vi "Write.vi"(8 "error in (no error)":errorcluster, 9 "Start address":string, 10 "Read Type":variant, 11 "MelsecTCP in":refnum<class "Abs Controler.lvclass">) -> (0 "error out":errorcluster, 3 "MelsecTCP out":refnum<class "Abs Controler.lvclass">)   [LabVIEW 2020, in "HslCommunication.lvlib" / "Abs Controler.lvclass"]
uses:
  Abs Controler.lvclass
  E:/Git/Libraries/develop/HslCommunication/_Dependenciecs/HslCommunication.dll
  _Dependenciecs/HslCommunication.dll
  <vilib>/Utility/Data Type/NI_Data Type.lvlib
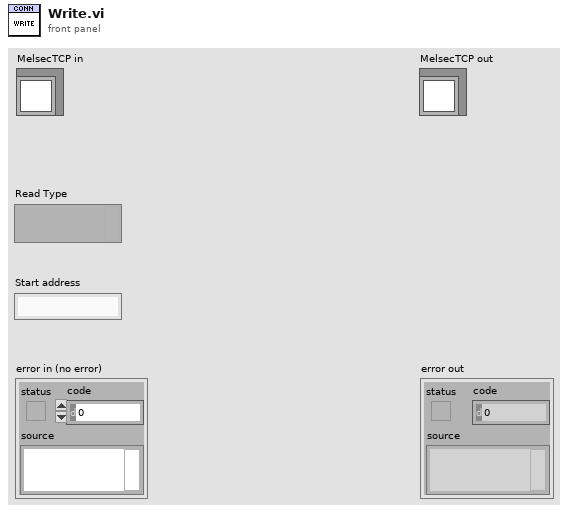
[diagram p1: front panel]
types:
  T1 = typedef "NI_Data Type.lvlib/Data Type.ctl" = enum8{"Invalid Type", "Void", "I8", "I16", "I32", "I64", "U8", "U16", "U32", "U64", "Single Float", "Double Float", "Extended Float", "Single Complex", "Double Complex", "Extended Complex", "Enum U8", "Enum U16", "Enum U32", "Enum U64", "Single Float With Unit", "Double Float With Unit", "Extended Float With Unit", "Single Complex with Unit", "Double Complex with Unit", "Extended Complex with Unit", "Boolean", "String", "Path", "Picture", "Tag", "Array", "Cluster", "Variant", "LV Variant", "Waveform", "Timestamp", "Digital Waveform", "Digital Data", "ExpressData", "Refnum", "External Data", "VI", "Poly VI", "LabVIEW Class Instance", "Fixed Point", "Set Collection", "Map Collection"}
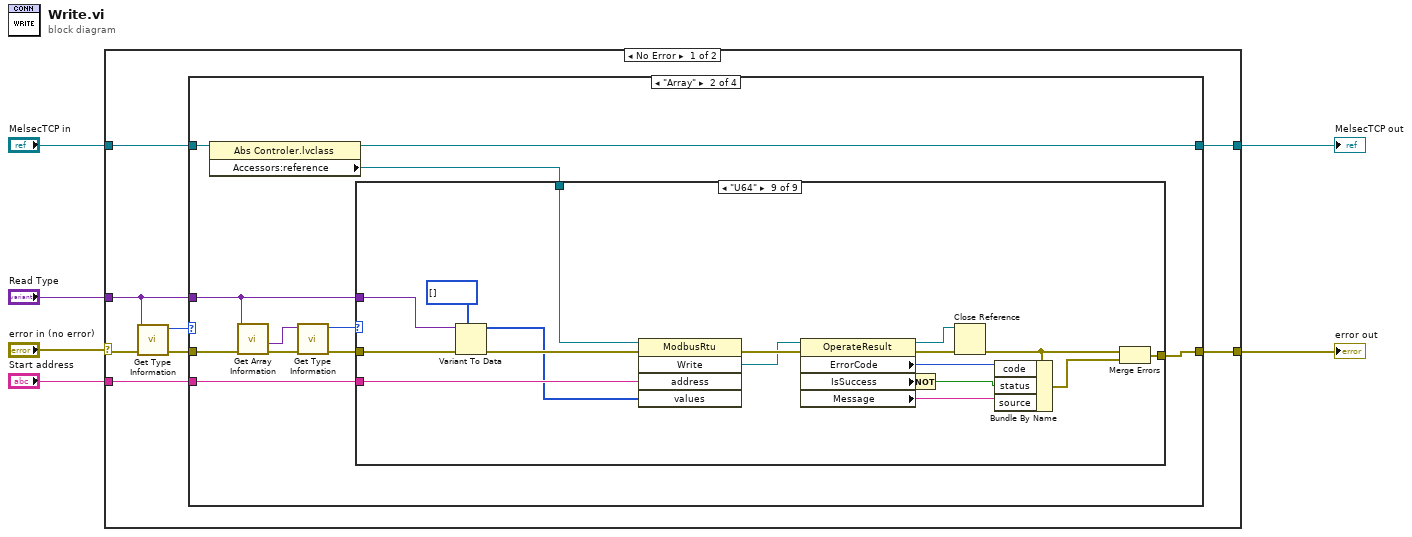
[diagram p0: block diagram]
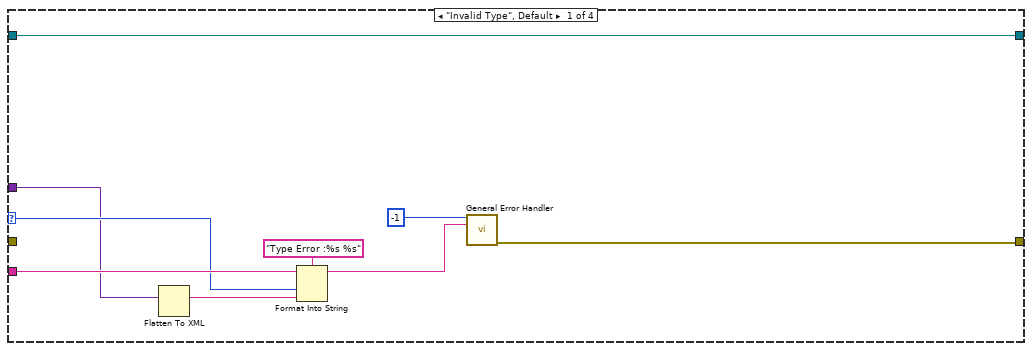
[diagram p2: hidden frame]
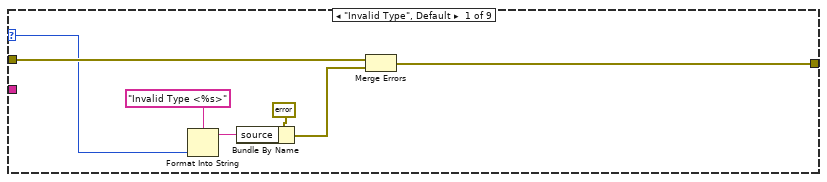
[diagram p3: hidden frame]
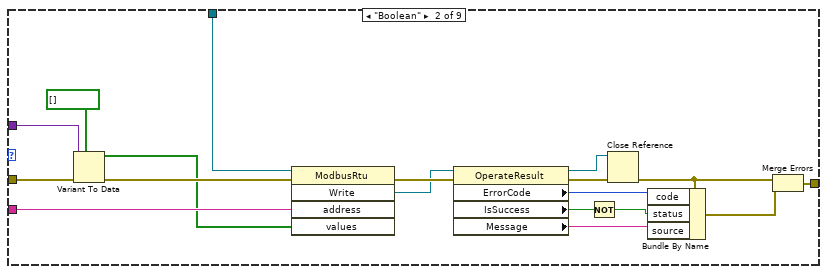
[diagram p4: hidden frame]
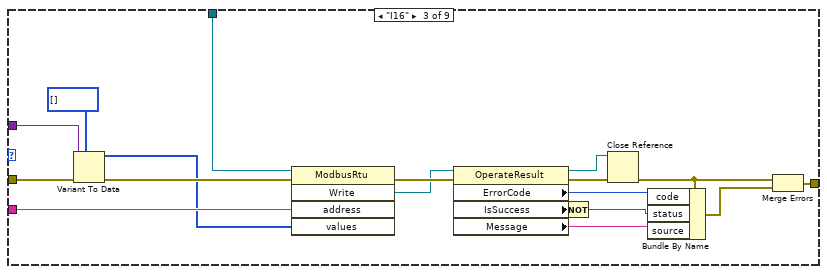
[diagram p5: hidden frame]
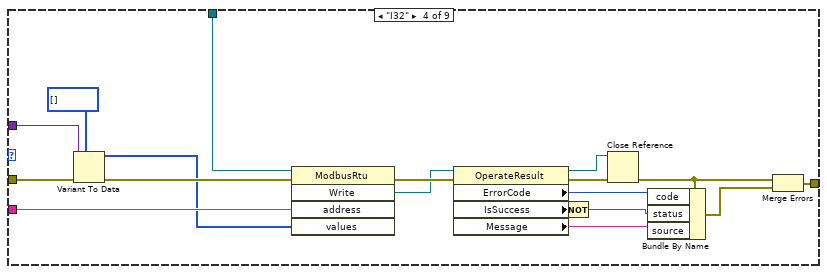
[diagram p6: hidden frame]
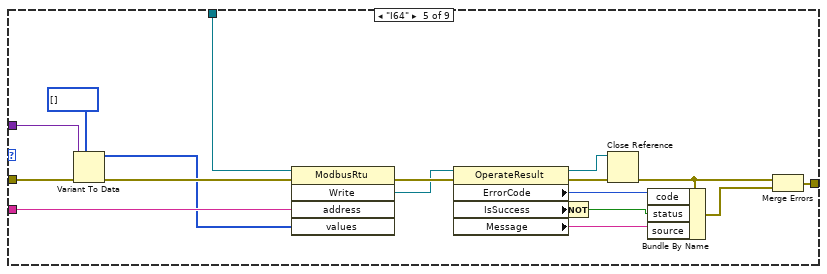
[diagram p7: hidden frame]
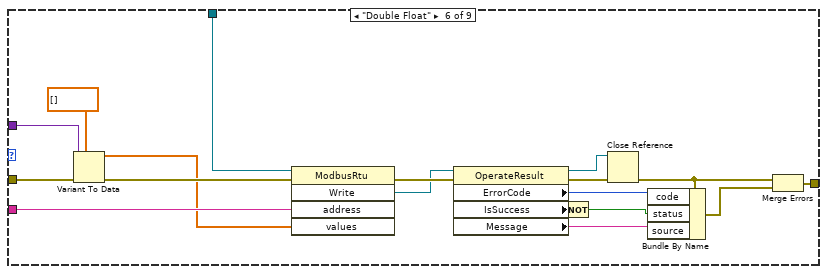
[diagram p8: hidden frame]
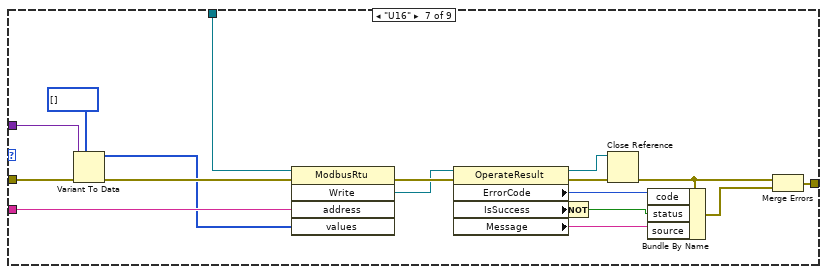
[diagram p9: hidden frame]
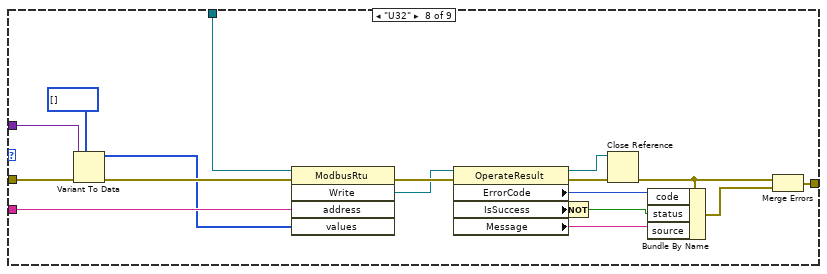
[diagram p10: hidden frame]
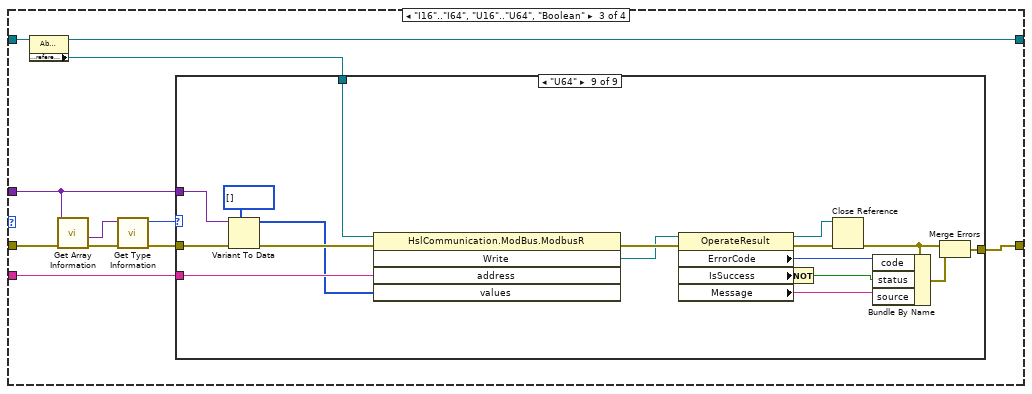
[diagram p11: hidden frame]
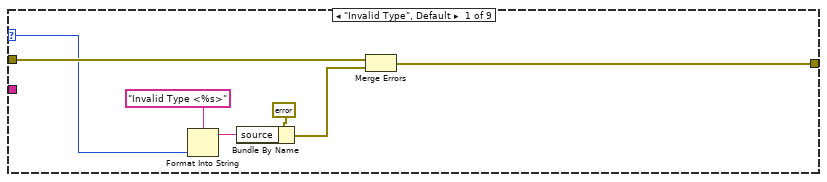
[diagram p12: hidden frame]
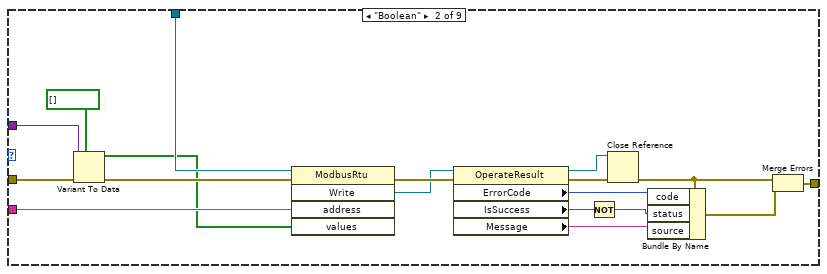
[diagram p13: hidden frame]
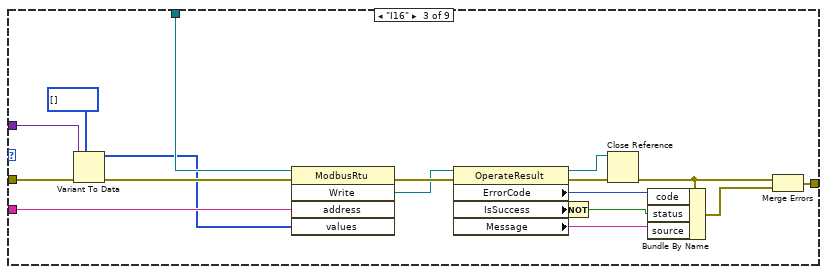
[diagram p14: hidden frame]
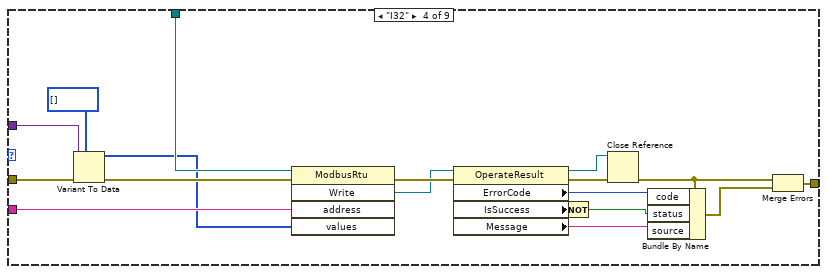
[diagram p15: hidden frame]
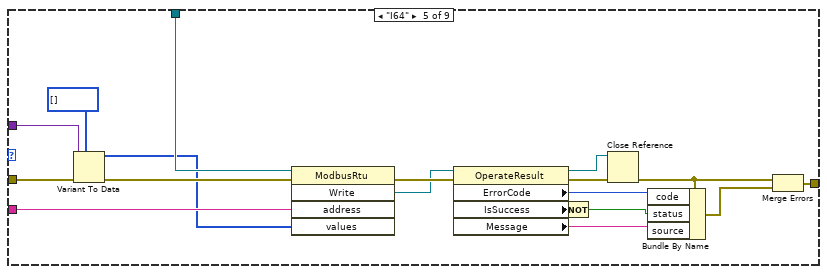
[diagram p16: hidden frame]
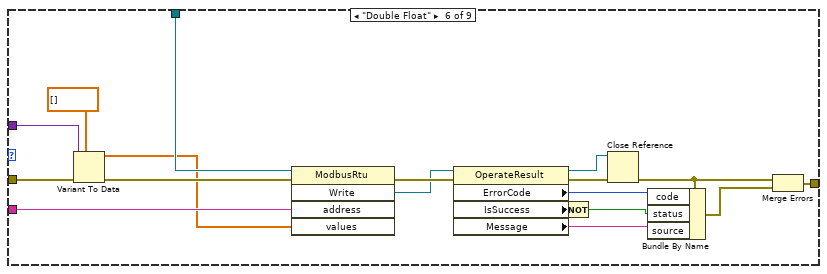
[diagram p17: hidden frame]
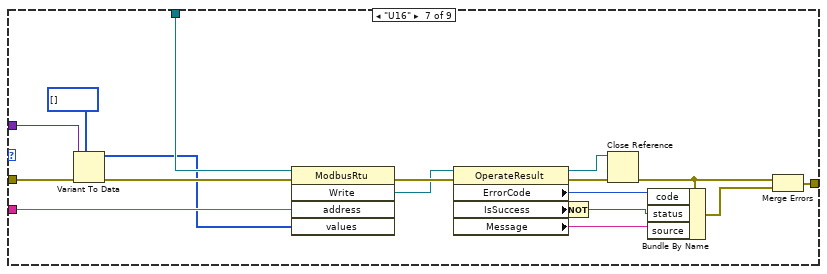
[diagram p18: hidden frame]
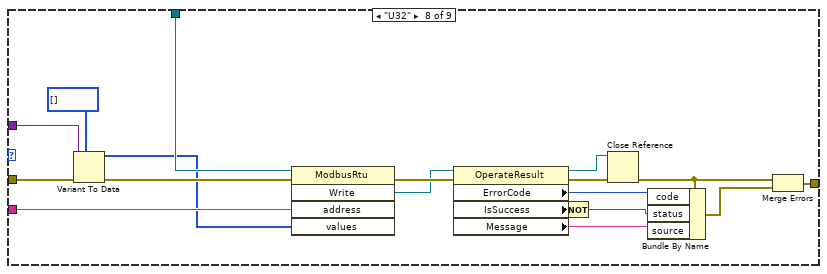
[diagram p19: hidden frame]
diagram:
  n1 = case shown="No Error" "error in (no error)" {
    selector: "error in (no error)" -> [w10 w351]
    tunnel: "MelsecTCP in" -> [w13 w350]
    tunnel: [w14 w350] -> w1
    tunnel: "Start address" -> [w12 _]
    tunnel: [w11 w351] -> w3
    tunnel: "Read Type" -> [w7 _]
    frame No Error {
      n2 = call <vilib>:"Get Type Information.vi"("error in (no error)"=w10, "variant"=w7) -> ("error out"=w9:errorcluster, "type"=w8:T1)  [unwired: 5 in, 3 out]
      n3 = case shown="\"Array\"" w8 {
        selector: w8 -> [w17 _ _ _]
        tunnel: [w23 w33 w195 w349] -> w14
        tunnel: w13 -> [w23 w28 w190 w349]
        tunnel: w9 -> [_ w27 w189 w348]
        tunnel: w12 -> [w19 w26 w188 _]
        tunnel: w7 -> [w16 w25 w187 _]
        tunnel: [w22 w24 w186 w348] -> w11
        frame "Invalid Type", Default {
          n4 = Flatten To XML(6:w16) -> (2:w15:string)
          n5 = Format Into String(format string="Type Error :%s %s", initial string=w19, w17, w15) -> (resulting string=w20:string)  [unwired: 1 in, 1 out]
          n6 = call <vilib>:"General Error Handler.vi"("[error code] (0)"=-1, "[error source] (\" \")"=w20) -> ("error out"=w22:errorcluster)  [unwired: 9 in, 4 out]
        }
        frame "Array" {
          n7 = property class="Abs Controler.lvclass"(reference=w28) -> (reference out=w33:refnum<class "Abs Controler.lvclass">, "Accessors:reference"=w34:refnum<k24>)  [unwired: 1 in, 1 out]
          n8 = call <vilib>:"Get Array Information.vi"("error in (no error)"=w27, "variant"=w25) -> ("error out"=w31:errorcluster, "array element data type"=w32:variant)  [unwired: 6 in, 2 out]
          n9 = call <vilib>:"Get Type Information.vi"("error in (no error)"=w31, "variant"=w32) -> ("error out"=w30:errorcluster, "type"=w29:T1)  [unwired: 5 in, 3 out]
          n10 = case shown="\"U64\"" w29 {
            selector: w29 -> [w39 _ _ _ _ _ _ _ _]
            tunnel: w34 -> [_ w59 w77 w95 w113 w131 w149 w167 w185]
            tunnel: w26 -> [_ w58 w76 w94 w112 w130 w148 w166 w184]
            tunnel: [w40 w57 w75 w93 w111 w129 w147 w165 w183] -> w24
            tunnel: w25 -> [_ w51 w69 w87 w105 w123 w141 w159 w177]
            tunnel: w30 -> [w41 w50 w68 w86 w104 w122 w140 w158 w176]
            frame "Invalid Type", Default {
              n11 = Format Into String(format string="Invalid Type <%s>", w39) -> (resulting string=w36:string)  [unwired: 2 in, 1 out]
              n12 = Bundle By Name(cluster=errorcluster {"status"=TRUE, "code"=-1, "source"=""} ("error IO"), "source"=w36) -> (w35:errorcluster)
              n13 = Merge Errors(w41, w35) -> (w40:errorcluster)
            }
            frame "Boolean" {
              n14 = Variant To Data(error in=w50, type=bool[] [], Variant=w51) -> (data=w43:bool[], error out=w45:errorcluster)
              n15 = invoke class="ModbusRtu" method="Write"(reference=w59, error in=w45, "address"=w58, "values"=w43) -> (error out=w49:errorcluster, "Write"=w47:refnum<k24>)  [unwired: 1 in, 3 out]
              n16 = property class="OperateResult"(reference=w47, error in=w49) -> (reference out=w46:refnum<k24>, error out=w48:errorcluster, "ErrorCode"=w56:i32, "IsSuccess"=w55:bool, "Message"=w54:string)
              n17 = Not(x=w55) -> (.not. x?=w42:bool)
              n18 = Close Reference(reference=w46, error in (no error)=w48) -> (error out=w53:errorcluster)
              n19 = Bundle By Name(cluster=w53, "code"=w56, "status"=w42, "source"=w54) -> (w52:errorcluster)
              n20 = Merge Errors(w53, w52) -> (w57:errorcluster)
            }
            frame "I16" {
              n21 = Variant To Data(error in=w68, type=i16[] [], Variant=w69) -> (data=w61:i16[], error out=w63:errorcluster)
              n22 = invoke class="ModbusRtu" method="Write"(reference=w77, error in=w63, "address"=w76, "values"=w61) -> (error out=w67:errorcluster, "Write"=w65:refnum<k24>)  [unwired: 1 in, 3 out]
              n23 = property class="OperateResult"(reference=w65, error in=w67) -> (reference out=w64:refnum<k24>, error out=w66:errorcluster, "ErrorCode"=w74:i32, "IsSuccess"=w73:bool, "Message"=w72:string)
              n24 = Not(x=w73) -> (.not. x?=w60:bool)
              n25 = Close Reference(reference=w64, error in (no error)=w66) -> (error out=w71:errorcluster)
              n26 = Bundle By Name(cluster=w71, "code"=w74, "status"=w60, "source"=w72) -> (w70:errorcluster)
              n27 = Merge Errors(w71, w70) -> (w75:errorcluster)
            }
            frame "I32" {
              n28 = Variant To Data(error in=w86, type=i32[] [], Variant=w87) -> (data=w79:i32[], error out=w81:errorcluster)
              n29 = invoke class="ModbusRtu" method="Write"(reference=w95, error in=w81, "address"=w94, "values"=w79) -> (error out=w85:errorcluster, "Write"=w83:refnum<k24>)  [unwired: 1 in, 3 out]
              n30 = property class="OperateResult"(reference=w83, error in=w85) -> (reference out=w82:refnum<k24>, error out=w84:errorcluster, "ErrorCode"=w92:i32, "IsSuccess"=w91:bool, "Message"=w90:string)
              n31 = Not(x=w91) -> (.not. x?=w78:bool)
              n32 = Close Reference(reference=w82, error in (no error)=w84) -> (error out=w89:errorcluster)
              n33 = Bundle By Name(cluster=w89, "code"=w92, "status"=w78, "source"=w90) -> (w88:errorcluster)
              n34 = Merge Errors(w89, w88) -> (w93:errorcluster)
            }
            frame "I64" {
              n35 = Variant To Data(error in=w104, type=i64[] [], Variant=w105) -> (data=w97:i64[], error out=w99:errorcluster)
              n36 = invoke class="ModbusRtu" method="Write"(reference=w113, error in=w99, "address"=w112, "values"=w97) -> (error out=w103:errorcluster, "Write"=w101:refnum<k24>)  [unwired: 1 in, 3 out]
              n37 = property class="OperateResult"(reference=w101, error in=w103) -> (reference out=w100:refnum<k24>, error out=w102:errorcluster, "ErrorCode"=w110:i32, "IsSuccess"=w109:bool, "Message"=w108:string)
              n38 = Not(x=w109) -> (.not. x?=w96:bool)
              n39 = Close Reference(reference=w100, error in (no error)=w102) -> (error out=w107:errorcluster)
              n40 = Bundle By Name(cluster=w107, "code"=w110, "status"=w96, "source"=w108) -> (w106:errorcluster)
              n41 = Merge Errors(w107, w106) -> (w111:errorcluster)
            }
            frame "Double Float" {
              n42 = Variant To Data(error in=w122, type=dbl[] [], Variant=w123) -> (data=w115:dbl[], error out=w117:errorcluster)
              n43 = invoke class="ModbusRtu" method="Write"(reference=w131, error in=w117, "address"=w130, "values"=w115) -> (error out=w121:errorcluster, "Write"=w119:refnum<k24>)  [unwired: 1 in, 3 out]
              n44 = property class="OperateResult"(reference=w119, error in=w121) -> (reference out=w118:refnum<k24>, error out=w120:errorcluster, "ErrorCode"=w128:i32, "IsSuccess"=w127:bool, "Message"=w126:string)
              n45 = Not(x=w127) -> (.not. x?=w114:bool)
              n46 = Close Reference(reference=w118, error in (no error)=w120) -> (error out=w125:errorcluster)
              n47 = Bundle By Name(cluster=w125, "code"=w128, "status"=w114, "source"=w126) -> (w124:errorcluster)
              n48 = Merge Errors(w125, w124) -> (w129:errorcluster)
            }
            frame "U16" {
              n49 = Variant To Data(error in=w140, type=u16[] [], Variant=w141) -> (data=w133:u16[], error out=w135:errorcluster)
              n50 = invoke class="ModbusRtu" method="Write"(reference=w149, error in=w135, "address"=w148, "values"=w133) -> (error out=w139:errorcluster, "Write"=w137:refnum<k24>)  [unwired: 1 in, 3 out]
              n51 = property class="OperateResult"(reference=w137, error in=w139) -> (reference out=w136:refnum<k24>, error out=w138:errorcluster, "ErrorCode"=w146:i32, "IsSuccess"=w145:bool, "Message"=w144:string)
              n52 = Not(x=w145) -> (.not. x?=w132:bool)
              n53 = Close Reference(reference=w136, error in (no error)=w138) -> (error out=w143:errorcluster)
              n54 = Bundle By Name(cluster=w143, "code"=w146, "status"=w132, "source"=w144) -> (w142:errorcluster)
              n55 = Merge Errors(w143, w142) -> (w147:errorcluster)
            }
            frame "U32" {
              n56 = Variant To Data(error in=w158, type=u32[] [], Variant=w159) -> (data=w151:u32[], error out=w153:errorcluster)
              n57 = invoke class="ModbusRtu" method="Write"(reference=w167, error in=w153, "address"=w166, "values"=w151) -> (error out=w157:errorcluster, "Write"=w155:refnum<k24>)  [unwired: 1 in, 3 out]
              n58 = property class="OperateResult"(reference=w155, error in=w157) -> (reference out=w154:refnum<k24>, error out=w156:errorcluster, "ErrorCode"=w164:i32, "IsSuccess"=w163:bool, "Message"=w162:string)
              n59 = Not(x=w163) -> (.not. x?=w150:bool)
              n60 = Close Reference(reference=w154, error in (no error)=w156) -> (error out=w161:errorcluster)
              n61 = Bundle By Name(cluster=w161, "code"=w164, "status"=w150, "source"=w162) -> (w160:errorcluster)
              n62 = Merge Errors(w161, w160) -> (w165:errorcluster)
            }
            frame "U64" {
              n63 = Variant To Data(error in=w176, type=u64[] [], Variant=w177) -> (data=w169:u64[], error out=w171:errorcluster)
              n64 = invoke class="ModbusRtu" method="Write"(reference=w185, error in=w171, "address"=w184, "values"=w169) -> (error out=w175:errorcluster, "Write"=w173:refnum<k24>)  [unwired: 1 in, 3 out]
              n65 = property class="OperateResult"(reference=w173, error in=w175) -> (reference out=w172:refnum<k24>, error out=w174:errorcluster, "ErrorCode"=w182:i32, "IsSuccess"=w181:bool, "Message"=w180:string)
              n66 = Not(x=w181) -> (.not. x?=w168:bool)
              n67 = Close Reference(reference=w172, error in (no error)=w174) -> (error out=w179:errorcluster)
              n68 = Bundle By Name(cluster=w179, "code"=w182, "status"=w168, "source"=w180) -> (w178:errorcluster)
              n69 = Merge Errors(w179, w178) -> (w183:errorcluster)
            }
          }
        }
        frame "I16".."I64", "U16".."U64", "Boolean" {
          n70 = property class="Abs Controler.lvclass"(reference=w190) -> (reference out=w195:refnum<class "Abs Controler.lvclass">, "Accessors:reference"=w196:refnum<k24>)  [unwired: 1 in, 1 out]
          n71 = call <vilib>:"Get Array Information.vi"("error in (no error)"=w189, "variant"=w187) -> ("error out"=w193:errorcluster, "array element data type"=w194:variant)  [unwired: 6 in, 2 out]
          n72 = call <vilib>:"Get Type Information.vi"("error in (no error)"=w193, "variant"=w194) -> ("error out"=w192:errorcluster, "type"=w191:T1)  [unwired: 5 in, 3 out]
          n73 = case shown="\"U64\"" w191 {
            selector: w191 -> [w201 _ _ _ _ _ _ _ _]
            tunnel: w196 -> [_ w221 w239 w257 w275 w293 w311 w329 w347]
            tunnel: w188 -> [_ w220 w238 w256 w274 w292 w310 w328 w346]
            tunnel: [w202 w219 w237 w255 w273 w291 w309 w327 w345] -> w186
            tunnel: w187 -> [_ w213 w231 w249 w267 w285 w303 w321 w339]
            tunnel: w192 -> [w203 w212 w230 w248 w266 w284 w302 w320 w338]
            frame "Invalid Type", Default {
              n74 = Format Into String(format string="Invalid Type <%s>", w201) -> (resulting string=w198:string)  [unwired: 2 in, 1 out]
              n75 = Bundle By Name(cluster=errorcluster {"status"=TRUE, "code"=-1, "source"=""} ("error IO"), "source"=w198) -> (w197:errorcluster)
              n76 = Merge Errors(w203, w197) -> (w202:errorcluster)
            }
            frame "Boolean" {
              n77 = Variant To Data(error in=w212, type=bool[] [], Variant=w213) -> (data=w205:bool[], error out=w207:errorcluster)
              n78 = invoke class="ModbusRtu" method="Write"(reference=w221, error in=w207, "address"=w220, "values"=w205) -> (error out=w211:errorcluster, "Write"=w209:refnum<k24>)  [unwired: 1 in, 3 out]
              n79 = property class="OperateResult"(reference=w209, error in=w211) -> (reference out=w208:refnum<k24>, error out=w210:errorcluster, "ErrorCode"=w218:i32, "IsSuccess"=w217:bool, "Message"=w216:string)
              n80 = Not(x=w217) -> (.not. x?=w204:bool)
              n81 = Close Reference(reference=w208, error in (no error)=w210) -> (error out=w215:errorcluster)
              n82 = Bundle By Name(cluster=w215, "code"=w218, "status"=w204, "source"=w216) -> (w214:errorcluster)
              n83 = Merge Errors(w215, w214) -> (w219:errorcluster)
            }
            frame "I16" {
              n84 = Variant To Data(error in=w230, type=i16[] [], Variant=w231) -> (data=w223:i16[], error out=w225:errorcluster)
              n85 = invoke class="ModbusRtu" method="Write"(reference=w239, error in=w225, "address"=w238, "values"=w223) -> (error out=w229:errorcluster, "Write"=w227:refnum<k24>)  [unwired: 1 in, 3 out]
              n86 = property class="OperateResult"(reference=w227, error in=w229) -> (reference out=w226:refnum<k24>, error out=w228:errorcluster, "ErrorCode"=w236:i32, "IsSuccess"=w235:bool, "Message"=w234:string)
              n87 = Not(x=w235) -> (.not. x?=w222:bool)
              n88 = Close Reference(reference=w226, error in (no error)=w228) -> (error out=w233:errorcluster)
              n89 = Bundle By Name(cluster=w233, "code"=w236, "status"=w222, "source"=w234) -> (w232:errorcluster)
              n90 = Merge Errors(w233, w232) -> (w237:errorcluster)
            }
            frame "I32" {
              n91 = Variant To Data(error in=w248, type=i32[] [], Variant=w249) -> (data=w241:i32[], error out=w243:errorcluster)
              n92 = invoke class="ModbusRtu" method="Write"(reference=w257, error in=w243, "address"=w256, "values"=w241) -> (error out=w247:errorcluster, "Write"=w245:refnum<k24>)  [unwired: 1 in, 3 out]
              n93 = property class="OperateResult"(reference=w245, error in=w247) -> (reference out=w244:refnum<k24>, error out=w246:errorcluster, "ErrorCode"=w254:i32, "IsSuccess"=w253:bool, "Message"=w252:string)
              n94 = Not(x=w253) -> (.not. x?=w240:bool)
              n95 = Close Reference(reference=w244, error in (no error)=w246) -> (error out=w251:errorcluster)
              n96 = Bundle By Name(cluster=w251, "code"=w254, "status"=w240, "source"=w252) -> (w250:errorcluster)
              n97 = Merge Errors(w251, w250) -> (w255:errorcluster)
            }
            frame "I64" {
              n98 = Variant To Data(error in=w266, type=i64[] [], Variant=w267) -> (data=w259:i64[], error out=w261:errorcluster)
              n99 = invoke class="ModbusRtu" method="Write"(reference=w275, error in=w261, "address"=w274, "values"=w259) -> (error out=w265:errorcluster, "Write"=w263:refnum<k24>)  [unwired: 1 in, 3 out]
              n100 = property class="OperateResult"(reference=w263, error in=w265) -> (reference out=w262:refnum<k24>, error out=w264:errorcluster, "ErrorCode"=w272:i32, "IsSuccess"=w271:bool, "Message"=w270:string)
              n101 = Not(x=w271) -> (.not. x?=w258:bool)
              n102 = Close Reference(reference=w262, error in (no error)=w264) -> (error out=w269:errorcluster)
              n103 = Bundle By Name(cluster=w269, "code"=w272, "status"=w258, "source"=w270) -> (w268:errorcluster)
              n104 = Merge Errors(w269, w268) -> (w273:errorcluster)
            }
            frame "Double Float" {
              n105 = Variant To Data(error in=w284, type=dbl[] [], Variant=w285) -> (data=w277:dbl[], error out=w279:errorcluster)
              n106 = invoke class="ModbusRtu" method="Write"(reference=w293, error in=w279, "address"=w292, "values"=w277) -> (error out=w283:errorcluster, "Write"=w281:refnum<k24>)  [unwired: 1 in, 3 out]
              n107 = property class="OperateResult"(reference=w281, error in=w283) -> (reference out=w280:refnum<k24>, error out=w282:errorcluster, "ErrorCode"=w290:i32, "IsSuccess"=w289:bool, "Message"=w288:string)
              n108 = Not(x=w289) -> (.not. x?=w276:bool)
              n109 = Close Reference(reference=w280, error in (no error)=w282) -> (error out=w287:errorcluster)
              n110 = Bundle By Name(cluster=w287, "code"=w290, "status"=w276, "source"=w288) -> (w286:errorcluster)
              n111 = Merge Errors(w287, w286) -> (w291:errorcluster)
            }
            frame "U16" {
              n112 = Variant To Data(error in=w302, type=u16[] [], Variant=w303) -> (data=w295:u16[], error out=w297:errorcluster)
              n113 = invoke class="ModbusRtu" method="Write"(reference=w311, error in=w297, "address"=w310, "values"=w295) -> (error out=w301:errorcluster, "Write"=w299:refnum<k24>)  [unwired: 1 in, 3 out]
              n114 = property class="OperateResult"(reference=w299, error in=w301) -> (reference out=w298:refnum<k24>, error out=w300:errorcluster, "ErrorCode"=w308:i32, "IsSuccess"=w307:bool, "Message"=w306:string)
              n115 = Not(x=w307) -> (.not. x?=w294:bool)
              n116 = Close Reference(reference=w298, error in (no error)=w300) -> (error out=w305:errorcluster)
              n117 = Bundle By Name(cluster=w305, "code"=w308, "status"=w294, "source"=w306) -> (w304:errorcluster)
              n118 = Merge Errors(w305, w304) -> (w309:errorcluster)
            }
            frame "U32" {
              n119 = Variant To Data(error in=w320, type=u32[] [], Variant=w321) -> (data=w313:u32[], error out=w315:errorcluster)
              n120 = invoke class="ModbusRtu" method="Write"(reference=w329, error in=w315, "address"=w328, "values"=w313) -> (error out=w319:errorcluster, "Write"=w317:refnum<k24>)  [unwired: 1 in, 3 out]
              n121 = property class="OperateResult"(reference=w317, error in=w319) -> (reference out=w316:refnum<k24>, error out=w318:errorcluster, "ErrorCode"=w326:i32, "IsSuccess"=w325:bool, "Message"=w324:string)
              n122 = Not(x=w325) -> (.not. x?=w312:bool)
              n123 = Close Reference(reference=w316, error in (no error)=w318) -> (error out=w323:errorcluster)
              n124 = Bundle By Name(cluster=w323, "code"=w326, "status"=w312, "source"=w324) -> (w322:errorcluster)
              n125 = Merge Errors(w323, w322) -> (w327:errorcluster)
            }
            frame "U64" {
              n126 = Variant To Data(error in=w338, type=u64[] [], Variant=w339) -> (data=w331:u64[], error out=w333:errorcluster)
              n127 = invoke class="HslCommunication.ModBus.ModbusR" method="Write"(reference=w347, error in=w333, "address"=w346, "values"=w331) -> (error out=w337:errorcluster, "Write"=w335:refnum<k24>)  [unwired: 1 in, 3 out]
              n128 = property class="OperateResult"(reference=w335, error in=w337) -> (reference out=w334:refnum<k24>, error out=w336:errorcluster, "ErrorCode"=w344:i32, "IsSuccess"=w343:bool, "Message"=w342:string)
              n129 = Not(x=w343) -> (.not. x?=w330:bool)
              n130 = Close Reference(reference=w334, error in (no error)=w336) -> (error out=w341:errorcluster)
              n131 = Bundle By Name(cluster=w341, "code"=w344, "status"=w330, "source"=w342) -> (w340:errorcluster)
              n132 = Merge Errors(w341, w340) -> (w345:errorcluster)
            }
          }
        }
        frame "Void" {
        }
      }
    }
    frame Error {
    }
  }
  "error out" <- w3
  "MelsecTCP out" <- w1
